vi "DOF 2 Group Text & Index.vi"(10 "IsCommand":bool, 11 "DOF Vector":T1(ring)) -> (1 "IsForce":bool, 2 "DOF Index":u32, 3 "Cart Channel Group Text":string)   [LabVIEW 2013]
uses:
  Space Group Type.ctl
  Cart Channel  Group Type.ctl
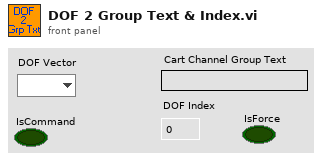
[diagram p1: front panel]
types:
  T1 = enum16{" ", "Dx", "Dy", "Dz", "Rx", "Ry", "Rz", "Fx", "Fy", "Fz", "Mx", "My", "Mz"}
  T2 = typedef "Cart Channel  Group Type.ctl" = enum16{"Cmd", "Disp", "Load"}
  T3 = typedef "Space Group Type.ctl" = enum16{"Cart", "Act"}
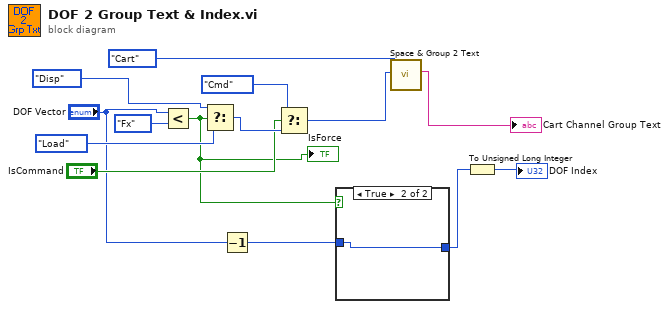
[diagram p0: block diagram]
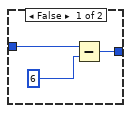
[diagram p2: hidden frame]
diagram:
  n1 = Less?(x="DOF Vector", y=T1."Fx") -> (x < y?=w1:bool)
  "IsForce" <- w1
  n2 = Select(t=Cart_Channel__Group_Type."Disp" ("Cart Channel Group Type"), s=w1, f=Cart_Channel__Group_Type."Load") -> (s? t:f=w10:T2)
  n3 = Decrement(x="DOF Vector") -> (x-1=w2:T1)
  n4 = Select(t=Cart_Channel__Group_Type."Cmd", s="IsCommand", f=w10) -> (s? t:f=w8:T2)
  n5 = case shown="True" w1 {
    tunnel: w2 -> [w17 w18]
    tunnel: [w15 w18] -> w3
    frame False {
      n6 = Subtract(x=w17, y=6) -> (x-y=w15:i32)
    }
    frame True {
    }
  }
  n7 = call "Space & Group 2 Text.vi"("Cart Channel Group Type"=w8, "Space Group Type"=Space_Group_Type."Cart") -> ("Text"=→"Cart Channel Group Text":string)  [unwired: 9 in]
  n8 = To Unsigned Long Integer(number=w3) -> (unsigned 32bit integer=→"DOF Index":u32)
